vi "Request Buffer.vi"(8 "error in (no error)":errorcluster, 11 "queue data in":T1={"server ID"=refnum, "Buffer data"={"decimation"=0, "avg bandwidth"=0.0, "channels"=[], "byte order"=enum."little-endian", "buffer descriptor"={"buffer type"=enum."Engine", "plugin id"=0, "group id"=0, "transfer id"=0, "offset"=0, "length"=0}, "values channels"={"index"=0, "count"=0, "engine offset"=0}, "select start offset"=18446744073709551615, "select end offset"=0, "channel index"=-1}} {"Buffer data"."channels"."configuration"."string offset" format="%d bytes"; "Buffer data"."avg bandwidth" format="%.0g bytes"}) -> (0 "error out":errorcluster, 3 "queue data out":T1={"server ID"=refnum, "Buffer data"={"decimation"=0, "avg bandwidth"=0.0, "channels"=[], "byte order"=enum."little-endian", "buffer descriptor"={"buffer type"=enum."Engine", "plugin id"=0, "group id"=0, "transfer id"=0, "offset"=0, "length"=0}, "values channels"={"index"=0, "count"=0, "engine offset"=0}, "select start offset"=18446744073709551615, "select end offset"=0, "channel index"=-1}} {"Buffer data"."channels"."configuration"."string offset" format="%d bytes"; "Buffer data"."avg bandwidth" format="%.0g bytes"})   [LabVIEW 2017, in "Data Viewer.lvlib"]
uses:
  Core/VIs/Data Viewer/Source/Data Viewer.lvlib
  Queue Data.ctl
  Buffer Data.ctl
  VeriStand/Data Sharing Custom Device/Source/DSF Core.lvlibp/Classes/Configuration/Core/Transfer/Channel Configuration.ctl
  VeriStand/Data Sharing Custom Device/Source/DSF Core.lvlibp/Typedefs/Core Channel Configuration.ctl
  VeriStand/Data Sharing Custom Device/Source/DSF Core.lvlibp/Typedefs/DSF Data Type.ctl
  VeriStand/Data Sharing Custom Device/Source/DSF Core.lvlibp/Typedefs/DSF Settings Info.ctl
  VeriStand/Data Sharing Custom Device/Source/DSF Core.lvlibp/Typedefs/DSF Byte Order.ctl
  VeriStand/Data Sharing Custom Device/Source/DSF Core.lvlibp/Classes/Thread/Data Server/DSF Buffer Subset Descriptor.ctl
  VeriStand/Data Sharing Custom Device/Source/DSF Core.lvlibp/Typedefs/DSF Buffer Type.ctl
  Main VI/Values Channels.ctl
  VeriStand/Data Sharing Custom Device/Source/DSF Core.lvlibp
  VeriStand/Data Sharing Custom Device/Source/DSF Core.lvlibp/Classes/Configuration/Core/Channel/Channel Configuration.lvclass
  VeriStand/Data Sharing Custom Device/Source/DSF Core.lvlibp/Classes/Configuration/Core/Transfer/Transfer Configuration.lvclass
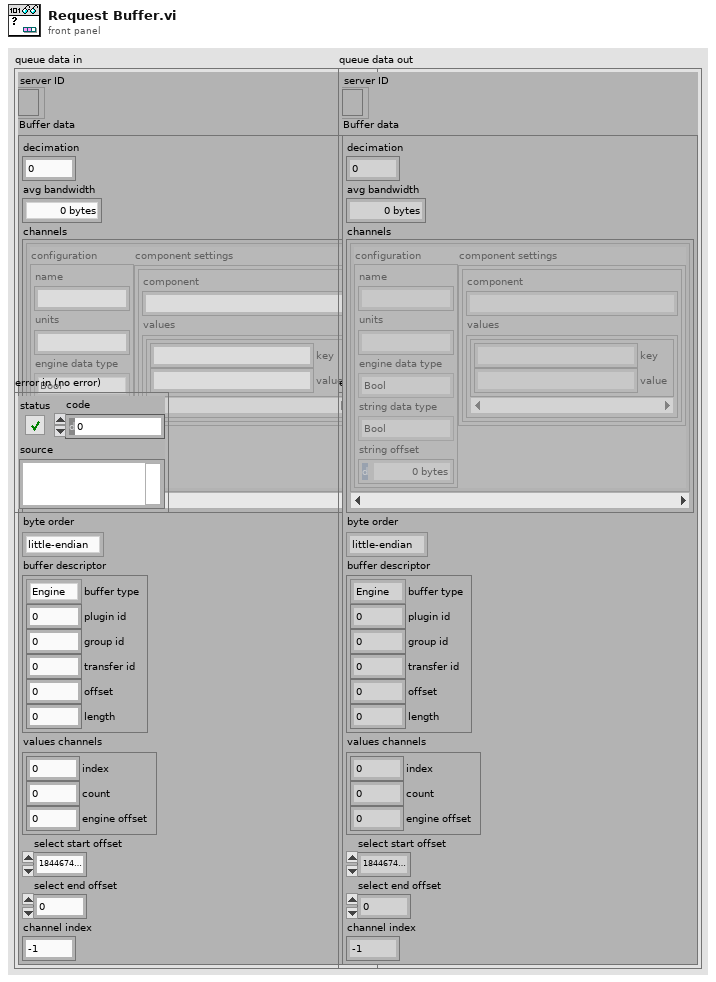
[diagram p1: front panel]
types:
  T1 = typedef "Data Viewer.lvlib/Queue Data.ctl" = cluster{"server ID":refnum<k5>, "Buffer data":T2}
  T2 = typedef "Data Viewer.lvlib/Buffer Data.ctl" = cluster{"decimation":u64, "avg bandwidth":dbl, "channels":T3[], "byte order":T7, "buffer descriptor":T8, "values channels":T10, "select start offset":u64, "select end offset":u64, "channel index":i32}
  T3 = typedef "DSF Core.lvlibp/Transfer Configuration.lvclass/Channel Configuration.ctl" = cluster{"configuration":T4, "component settings":T6[]}
  T4 = typedef "DSF Core.lvlibp/Channel Configuration.lvclass/Core Channel Configuration.ctl" = cluster{"name":string, "units":string, "engine data type":T5, "string data type":T5, "string offset":u64}
  T5 = typedef "DSF Core.lvlibp/DSF Data Type.ctl" = enum8{"Bool", "SGL", "DBL", "I8", "I16", "I32", "I64", "U8", "U16", "U32", "U64"}
  T6 = typedef "DSF Core.lvlibp/DSF Settings Info.ctl" = cluster{"component":string, "values":cluster{"key":string, "value":string}[]}
  T7 = typedef "DSF Core.lvlibp/DSF Byte Order.ctl" = enum8{"big-endian", "little-endian"}
  T8 = typedef "DSF Core.lvlibp/DSF Buffer Subset Descriptor.ctl" = cluster{"buffer type":T9, "plugin id":i32, "group id":i32, "transfer id":i32, "offset":u64, "length":i64}
  T9 = typedef "DSF Core.lvlibp/DSF Buffer Type.ctl" = enum16{"Engine", "String"}
  T10 = typedef "Data Viewer.lvlib/Values Channels.ctl" = cluster{"index":i32, "count":i32, "engine offset":u64}
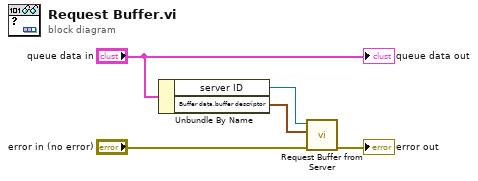
[diagram p0: block diagram]
diagram:
  n1 = Unbundle By Name("queue data in") -> ("server ID"=w1:refnum<k5>, "Buffer data.buffer descriptor"=w2:T8)
  n2 = call "Request Buffer from Server.vi"("error in (no error)"="error in (no error)", "buffer descriptor"=w2, "server ID in"=w1) -> ("error out"=→"error out":errorcluster)  [unwired: 6 in, 2 out]
  "queue data out" <- "queue data in"
